vi "getChannelByAddress.vi"(8 "error in (no error)":errorcluster, 10 "channel_address":string, 11 "ChannelArray in":refnum<class "ChannelArray.lvclass">) -> (0 "error out":errorcluster, 1 "found?":bool=TRUE, 2 "Channel":refnum<class "Channel.lvclass">, 3 "ChannelArray out":refnum<class "ChannelArray.lvclass">)   [LabVIEW 2009, in "Tools.lvlib" / "DatabaseHelpers.lvlib" / "ChannelArray.lvclass"]
uses:
  ChannelArray.lvclass
  Channel/Channel.lvclass
  ChannelArray.lvclass/ChannelArray.ctl
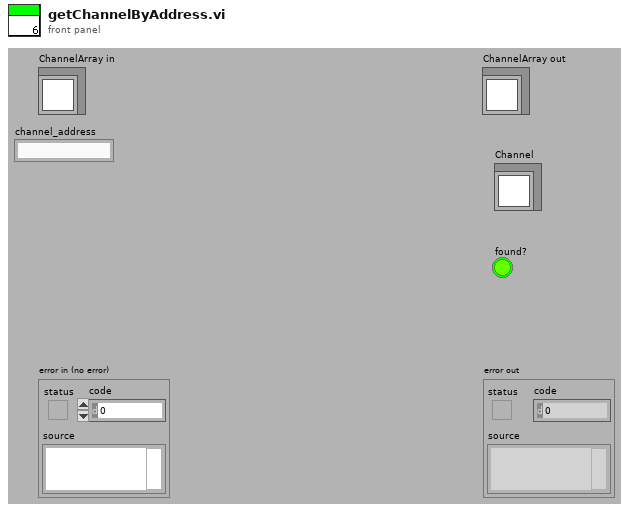
[diagram p1: front panel]
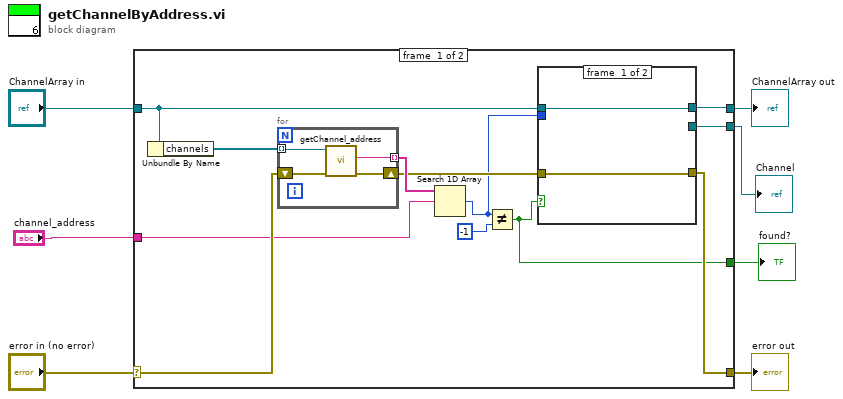
[diagram p0: block diagram]
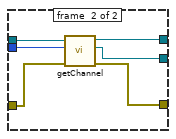
[diagram p2: hidden frame]
diagram:
  n1 = case shown="No Error" "error in (no error)" {
    selector: "error in (no error)" -> [w18 w33]
    tunnel: [w11 w33] -> w6
    tunnel: [w13 w32] -> w4
    tunnel: "ChannelArray in" -> [w14 w32]
    tunnel: "channel_address" -> [w16 _]
    tunnel: [w10 _] -> w2
    tunnel: [w8 _] -> w1
    frame #0 {
      n2 = Unbundle By Name(w14) -> ("channels"=w19:refnum<class "Channel.lvclass">[])
      n3 = for {
        tunnel: w19 -> [w31] mode=indexing
        tunnel: [w30] -> w17 mode=indexing
        shift-right: [w28] -> w12
        shift-left: w18 -> [w29]
        n4 = call "getChannel_address.vi"("error in (no error)"=w29, "Channel.lvclass in"=w31) -> ("error out"=w28:errorcluster, "channel_address"=w30:string)  [unwired: 7 in, 1 out]
      }
      n5 = Search 1D Array(1D array=w17, element=w16) -> (index of element=w9:i32)  [unwired: 1 in]
      n6 = Not Equal?(x=w9, y=-1) -> (x != y?=w10:bool)
      n7 = case shown="True" w10 {
        tunnel: w14 -> [w21 w27]
        tunnel: [w21 w26] -> w13
        tunnel: [w20 w25] -> w11
        tunnel: w12 -> [w20 w24]
        tunnel: w9 -> [_ w23]
        tunnel: [_ w22] -> w8
        frame #0 {
        }
        frame #1 {
          n8 = call "getChannel.vi"("error in (no error)"=w24, "index"=w23, "ChannelArray.lvclass in"=w27) -> ("error out"=w25:errorcluster, "Channel"=w22:refnum<class "Channel.lvclass">, "ChannelArray.lvclass out"=w26:refnum<class "ChannelArray.lvclass">)  [unwired: 6 in]
        }
      }
    }
    frame #1 {
    }
  }
  "error out" <- w6
  "ChannelArray out" <- w4
  "Channel" <- w1
  "found?" <- w2
